vi "trash_Error Global.vi"() -> ()   [LabVIEW 2021]
panel:
  in  "Long Sleep":errorcluster={"status"=FALSE, "code"=9002, "source"="The requested sleep deadline was greater than the configured maximum sleep.  If longer sleep times are typically needed raise the configured maximum sleep timer limit.  "}
  in  "Invalid ID":errorcluster={"status"=TRUE, "code"=9001, "source"="There is no active correlated clock for the provided input ID.  Check that the clock has been instantiated on the system.   "}
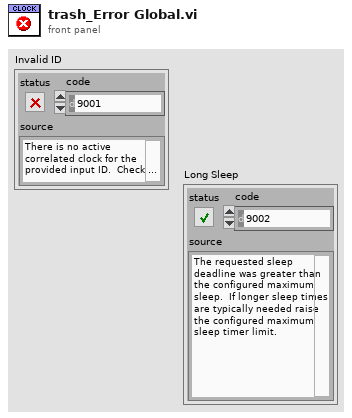
[diagram p1: front panel]
diagram:
